vi "Part 2.vi"(11 "Input":string) -> (3 "Output":i64)   [LabVIEW 2021]
uses:
  <userlib>/_OpenG.lib/string/string.llb/Convert EOLs (String)__ogtk.vi
panel:
  # "167409079868000"
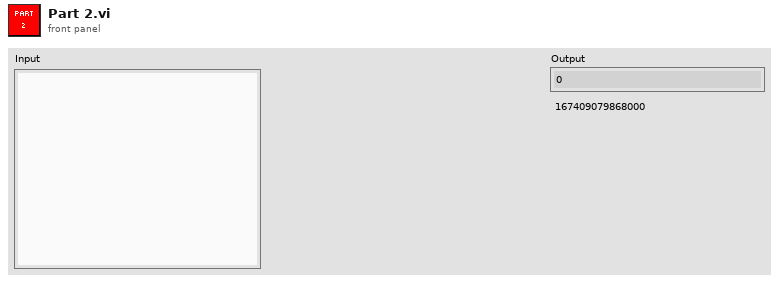
[diagram p1: front panel]
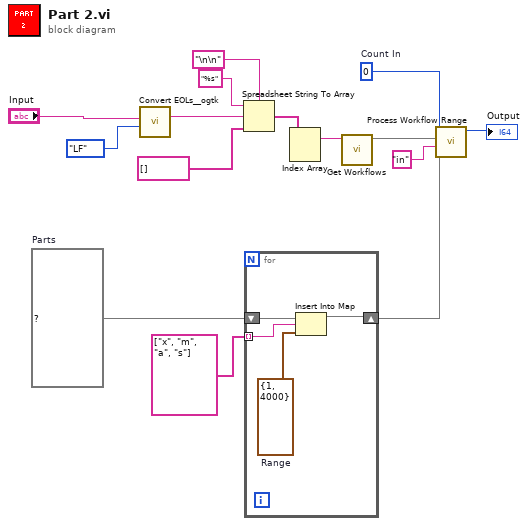
[diagram p0: block diagram]
diagram:
  w5 = i64 0  # Count In
  w7 = map{string, cluster{"Min":i64, "Max":i64}} {}  # Parts
  n1 = call-poly <userlib>:"Convert EOLs__ogtk.vi"("Convert to:"=enum16{"CR", "LF", "CRLF"}."LF", "String in"="Input") -> ("String out"=w11:string)  [unwired: 9 in]
  n2 = Spreadsheet String To Array(delimiter (Tab)="\n\n", format string="%s", spreadsheet string=w11, array type (2D Dbl)=string[] []) -> (array=w9:string[])
  n3 = for {
    shift-right: [w16] -> w2
    shift-left: w7 -> [w19]
    tunnel: string[] ["x", "m", "a", "s"] -> [w18] mode=indexing
    w17 = cluster{"Min":i64, "Max":i64} {"Min"=1, "Max"=4000}  # Range
    n4 = Insert Into Map(map in=w19, key=w18, value=w17) -> (map out=w16:map{string, cluster{"Min":i64, "Max":i64}})  [unwired: 2 out]
  }
  n5 = Index Array(array=w9) -> (element #1=w8:string)  [unwired: 2 in, 1 out]
  n6 = call "Get Workflows.vi"("Workflows In"=w8) -> ("Workflow Map"=w3:map{string, string[]})  [unwired: 10 in]
  n7 = call "Process Workflow Range.vi"("Parts"=w2, "Current Workflow"="in" ("delimiter (Tab)"), "Workflow Map"=w3, "Count In"=w5) -> ("Count Out"=→"Output":i64)  [unwired: 7 in]
